vi "Write lRMS.vi"(8 "error in (no error)":errorcluster, 10 "lRMS":dbl, 11 "PAS Cell Data in":refnum<class "PAS Cell Data.lvclass">) -> (0 "error out":errorcluster, 3 "PAS Cell Data out":refnum<class "PAS Cell Data.lvclass">)   [LabVIEW 2014, in "PAS Library.lvlib" / "PAS Cell Data.lvclass"]
uses:
  PAS Cell Data.lvclass
  PAS Cell Data.lvclass/PAS Cell Data.ctl
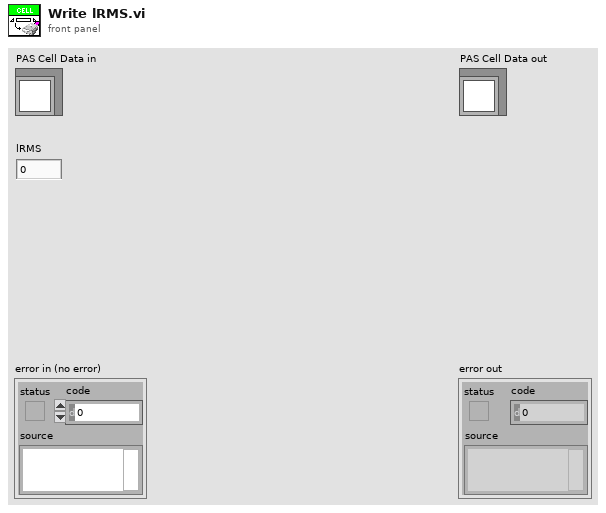
[diagram p1: front panel]
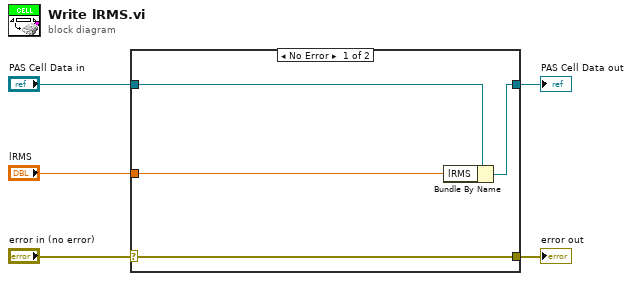
[diagram p0: block diagram]
diagram:
  n1 = case shown="No Error" "error in (no error)" {
    selector: "error in (no error)" -> [w9 w10]
    tunnel: [w9 w10] -> w4
    tunnel: [w7 w11] -> w2
    tunnel: "PAS Cell Data in" -> [w8 w11]
    tunnel: "lRMS" -> [w6 _]
    frame No Error {
      n2 = Bundle By Name(cluster=w8, "lRMS"=w6) -> (w7:refnum<class "PAS Cell Data.lvclass">)
    }
    frame Error {
    }
  }
  "error out" <- w4
  "PAS Cell Data out" <- w2
